vi "Time Global.vi"() -> ()   [LabVIEW 2019]
panel:
  in  "Turret":dbl=20.0
  in  "Drive":dbl=20.0
  in  "Intake":dbl=20.0
  in  "Indexer":dbl=20.0
  in  "Shooter":dbl=20.0
  in  "F.L.Y Stick Controller":dbl=20.0
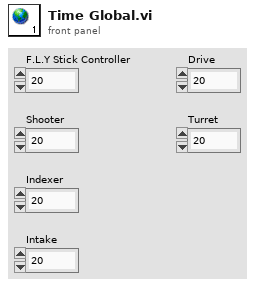
[diagram p1: front panel]
diagram:
